vi "globalcontrols.vi"() -> ()   [LabVIEW 2013]
panel:
  in  "Global Stop":bool
  in  "Global Switch":bool
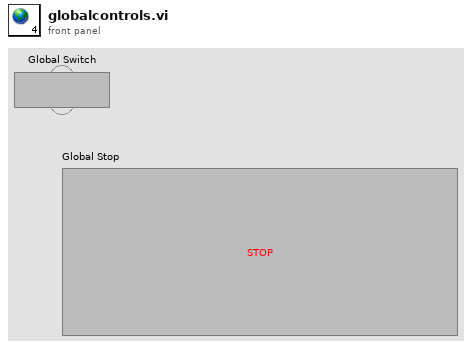
[diagram p1: front panel]
diagram:
